vi "Larger window send to front.vi"(9 "Image name":string, 11 "Window VI's Ref":refnum<vi>) -> ()   [LabVIEW 2013]
uses:
  Globals/gl_Time series viewer globals.vi
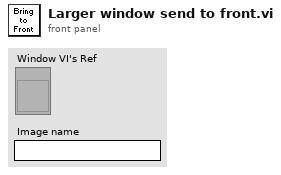
[diagram p1: front panel]
types:
  T1 = enum32{"Invalid", "Standard", "Closed", "Hidden", "Minimized", "Maximized"}
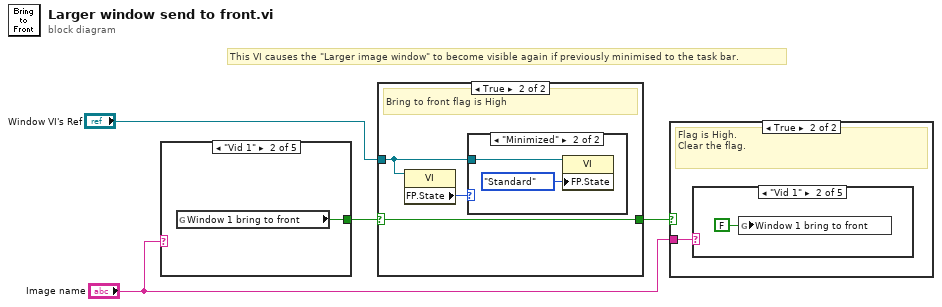
[diagram p0: block diagram]
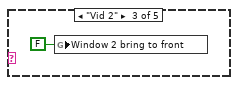
[diagram p4: hidden frame]
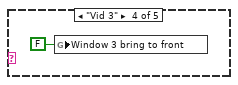
[diagram p5: hidden frame]
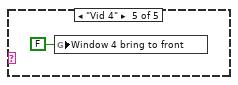
[diagram p6: hidden frame]
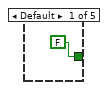
[diagram p9: hidden frame]
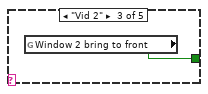
[diagram p10: hidden frame]
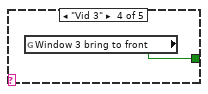
[diagram p11: hidden frame]
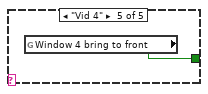
[diagram p12: hidden frame]
diagram:
  # "This VI causes the \"Larger image window\" to become visible again if previously minimised to the task bar."
  n1 = case shown="\"Vid 1\"" "Image name" {
    tunnel: [FALSE ("Window 4 bring to front") w6 w7 w8 w9] -> w3
    frame Default {
    }
    frame "Vid 1" {
      n2 = global read "gl_Time series viewer globals.vi" "Window 1 bring to front"() -> (w6:bool)
    }
    frame "Vid 2" {
      n3 = global read "gl_Time series viewer globals.vi" "Window 2 bring to front"() -> (w7:bool)
    }
    frame "Vid 3" {
      n4 = global read "gl_Time series viewer globals.vi" "Window 3 bring to front"() -> (w8:bool)
    }
    frame "Vid 4" {
      n5 = global read "gl_Time series viewer globals.vi" "Window 4 bring to front"() -> (w9:bool)
    }
  }
  n6 = case shown="True" w3 {
    selector: w3 -> [w10 w13]
    tunnel: [w10 w13] -> w4
    tunnel: "Window VI's Ref" -> [_ w12]
    frame False {
      # "Bring to front flag is Low"
    }
    frame True {
      # "Bring to front flag is High"
      n7 = property class="VI"(reference=w12) -> ("FP.State"=w11:T1)  [unwired: 1 in, 2 out]
      n8 = case shown="\"Minimized\"" w11 {
        tunnel: w12 -> [_ w15]
        frame Default {
        }
        frame "Minimized" {
          n9 = property class="VI"(reference=w15, "FP.State"=T1."Standard" ("Front Panel Window:State")) -> ()  [unwired: 1 in, 2 out]
        }
      }
    }
  }
  n10 = case shown="True" w4 {
    tunnel: "Image name" -> [_ w16]
    frame False {
      # "Flag is Low.\nDo nothing."
    }
    frame True {
      # "Flag is High. \nClear the flag."
      n11 = case shown="\"Vid 1\"" w16 {
        frame Default {
        }
        frame "Vid 1" {
          n12 = global write "gl_Time series viewer globals.vi" "Window 1 bring to front"(FALSE ("Window 1 bring to front")) -> ()
        }
        frame "Vid 2" {
          n13 = global write "gl_Time series viewer globals.vi" "Window 2 bring to front"(FALSE ("Window 2 bring to front")) -> ()
        }
        frame "Vid 3" {
          n14 = global write "gl_Time series viewer globals.vi" "Window 3 bring to front"(FALSE ("Window 3 bring to front")) -> ()
        }
        frame "Vid 4" {
          n15 = global write "gl_Time series viewer globals.vi" "Window 4 bring to front"(FALSE ("Window 4 bring to front")) -> ()
        }
      }
    }
  }
